vi "coerceData.vi"(9 "Eurotherm":T1) -> (1 "Eurotherm 2":T1)   [LabVIEW 2017]
panel:
  # "Coerce data.  ( A veces da lecturas sin sentido)"
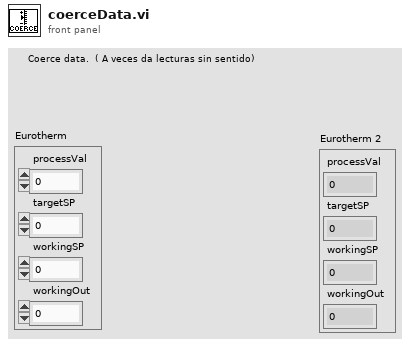
[diagram p1: front panel]
types:
  T1 = cluster{"processVal":dbl, "targetSP":dbl, "workingSP":dbl, "workingOut":dbl}
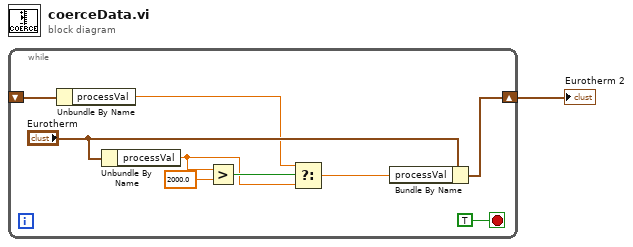
[diagram p0: block diagram]
diagram:
  n1 = while {
    shift-right: [w8] -> w1
    shift-left: _ -> [w5]
    stop <- TRUE stop-if-true
    n2 = Unbundle By Name(w5) -> ("processVal"=w4:dbl)
    n3 = Unbundle By Name("Eurotherm") -> ("processVal"=w3:dbl)
    n4 = Greater?(x=w3, y=2000.0) -> (0:w6:bool)
    n5 = Select(t=w4, s=w6, f=w3) -> (s? t:f=w2:dbl)
    n6 = Bundle By Name(cluster="Eurotherm", "processVal"=w2) -> (w8:T1)
  }
  "Eurotherm 2" <- w1
